vi "generate polar angle distribution start.vi"(1 "speed of light [m/s]":sgl=300000000.0, 5 "position c events":T1[](array[typedef]), 6 "position b events":T1[](array[typedef]), 7 "position a events":T1[](array[typedef]), 8 "origin events":T1[](array[typedef])) -> (0 "number of viable source locations":i32, 2 "polar angle distibution array":T2[](array[typedef]), 3 "polar xy graph cluster":cluster{sgl[], sgl[]})   [LabVIEW 2014]
doc: "This subVI should calculate the components of the unit vectors to all of the possible sources from the given event data distributions from each sensor. It then should calculate the 3D polar angles from the 3D unit vectors. It should ouput an array of possible source locations and a polar plot of the entire distibution."
uses:
  F:/All_Physics/PHY_350/Assignments/E4 R 1-28 to R 2-4/E4 start/typedefs/polar angle typedef.ctl
  F:/All_Physics/PHY_350/Assignments/E4 R 1-28 to R 2-4/E4 start/typedefs/event cluster typedef.ctl
  F:/All_Physics/PHY_350/Assignments/E4 R 1-28 to R 2-4/E4 start/typedefs/unit vector typedef.ctl
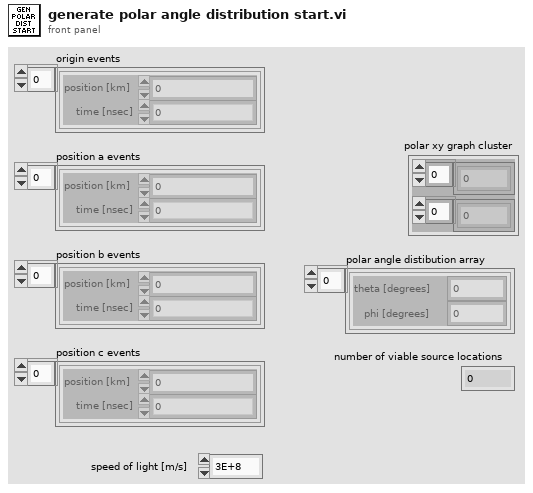
[diagram p1: front panel]
types:
  T1 = typedef "event cluster typedef.ctl" = cluster{"position [km]":sgl, "time [nsec]":i64}
  T2 = typedef "polar angle typedef.ctl" = cluster{"theta [degrees]":sgl, "phi [degrees]":sgl}
  T3 = typedef "unit vector typedef.ctl" = cluster{"nx":sgl, "ny":sgl, "nz":sgl}
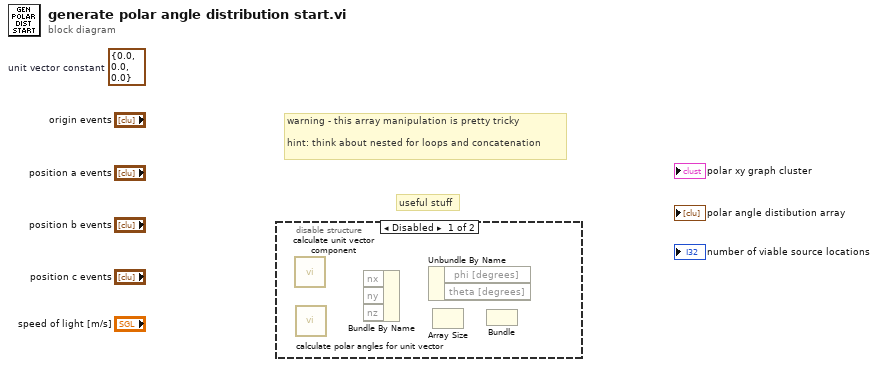
[diagram p0: block diagram]
diagram:
  (unwired) T3 {"nx"=0.0, "ny"=0.0, "nz"=0.0}  # unit vector constant
  # "warning - this array manipulation is pretty tricky\n\nhint: think about nested for loops and concatenation"
  # "useful stuff"
  n1 = disable-structure shown="Disabled" {
    frame Disabled {
      n2 = call "calculate unit vector component.vi"() -> ()  [unwired: 15 in, 1 out]
      n3 = call "calculate polar angles for unit vector.vi"() -> ()  [unwired: 13 in, 3 out]
      n4 = Bundle By Name() -> ()  [unwired: 4 in, 1 out]
      n5 = Unbundle By Name() -> ()  [unwired: 1 in, 2 out]
      n6 = Array Size() -> ()  [unwired: 1 in, 1 out]
      n7 = Bundle() -> ()  [unwired: 3 in, 1 out]
    }
    frame Enabled {
    }
  }
